vi "StopAsyncEngine.vi"(8 "error in (no error)":errorcluster, 11 "MicronGRPCClient in":refnum<class "MicronGRPCClient.lvclass">) -> (0 "error out":errorcluster, 3 "MicronGRPCClient out":refnum<class "MicronGRPCClient.lvclass">)   [LabVIEW 2019, in "MicronGRPCClient.lvclass"]
uses:
  MicronGRPCClient.lvclass
  MicronGRPCClient.lvclass/MicronGRPCClient.ctl
  66b8622b-e549-4d13-b040-40250e5ace5e.vi
  <vilib>/SLL Toolkit/SLL Queued State Machine/Queue Driver/Enqueue an Item to Queue.vi
  <vilib>/SLL Toolkit/SLL Queued State Machine/Queue Driver/Flush Queue.vi
  <vilib>/SLL Toolkit/SLL Queued State Machine/Queue Driver/Release Queue.vi
  <vilib>/SLL Toolkit/SLL Queued State Machine/SLL QSM.lvlib
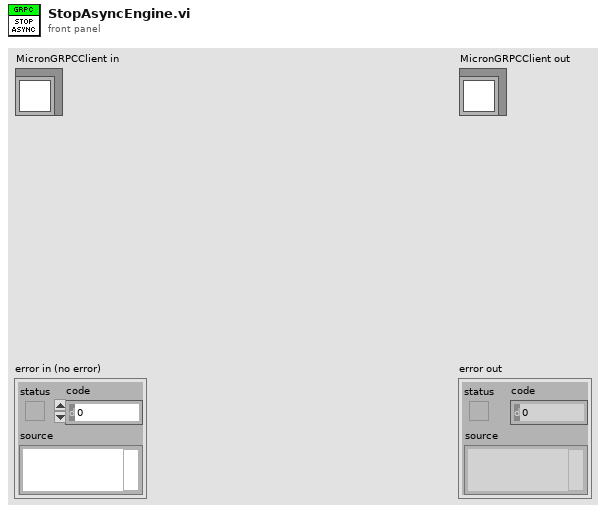
[diagram p1: front panel]
types:
  T1 = typedef "MicronGRPCClient.lvclass/AsyncCluster.ctl" = cluster{"InputQueue":refnum<queue>, "OutputQueue":refnum<queue>}
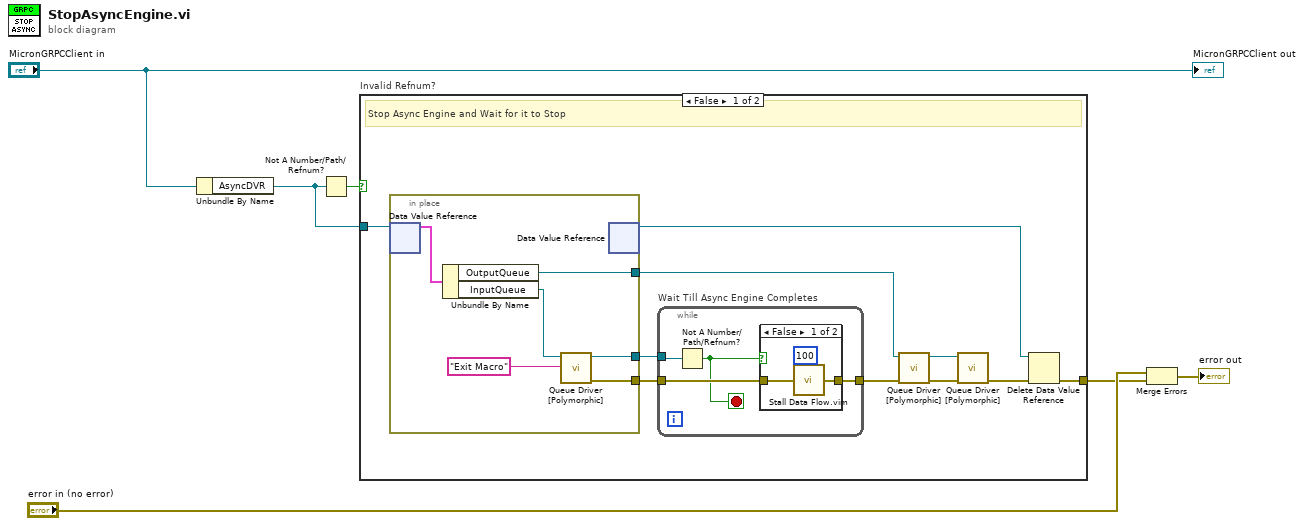
[diagram p0: block diagram]
diagram:
  n1 = Unbundle By Name("MicronGRPCClient in") -> ("AsyncDVR"=w4:refnum<data-value>)
  n2 = Not A Number/Path/Refnum?(number/path/refnum=w4) -> (NaN/Path/Refnum?=w5:bool)
  n3 = case "Invalid Refnum?" shown="False" w5 {
    tunnel: w4 -> [w16 _]
    tunnel: [w15 _] -> w1
    frame False {
      # "Stop Async Engine and Wait for it to Stop"
      n4 = in-place {
        in-place-border: [w27] -> w11
        in-place-border: [w26] -> w13
        in-place-border: [w25] -> w12
        n5 = in-place-dvr #1(w16) -> (w30:T1)  [unwired: 1 out]
        n6 = Unbundle By Name(w30) -> ("OutputQueue"=w26:refnum<queue>, "InputQueue"=w29:refnum<queue>)
        n7 = call-poly <vilib>:"Queue Driver [Polymorphic].vi"("Item to Add"="Exit Macro", "Queue Ref In"=w29) -> ("Error Out"=w27:errorcluster, "Queue Ref Out"=w25:refnum<queue>)  [unwired: 8 in]
        n8 = in-place-dvr #1() -> (w14:refnum<data-value>)  [unwired: 1 in, 1 out]
      }
      n9 = while "Wait Till Async Engine Completes" {
        tunnel: w12 -> [w20]
        tunnel: w11 -> [w19]
        tunnel: [w18] -> w10
        stop <- w17 stop-if-true
        n10 = Not A Number/Path/Refnum?(number/path/refnum=w20) -> (NaN/Path/Refnum?=w17:bool)
        n11 = case shown="False" w17 {
          tunnel: w19 -> [w23 w24]
          tunnel: [w22 w24] -> w18
          frame False {
            n12 = call "Stall Data Flow.vim"("value in"=w23, "milliseconds to wait"=u32 100) -> ("value out"=w22:errorcluster)  [unwired: 1 out]
          }
          frame True {
          }
        }
      }
      n13 = call-poly <vilib>:"Queue Driver [Polymorphic].vi"("Error In"=w10, "Queue Ref In"=w13) -> ("Error Out"=w8:errorcluster, "Queue Ref Out"=w9:refnum<queue>)  [unwired: 7 in, 1 out]
      n14 = call-poly <vilib>:"Queue Driver [Polymorphic].vi"("Error In"=w8, "Queue Ref In"=w9) -> ("Error Out"=w7:errorcluster)  [unwired: 9 in]
      n15 = Delete Data Value Reference(data value reference=w14, error in=w7) -> (error out=w15:errorcluster)  [unwired: 1 out]
    }
    frame True {
      # "No Action Needed"
    }
  }
  n16 = Merge Errors("error in (no error)", w1) -> (→"error out":errorcluster)
  "MicronGRPCClient out" <- "MicronGRPCClient in"
